vi "set_power.vi"(8 "error in (no error)":errorcluster, 10 "Power":sgl=100.0, 11 "Laser_Ethernet in":refnum<class "Laser_Ethernet.lvclass">) -> (0 "error out":errorcluster, 3 "Laser_Ethernet out":refnum<class "Laser_Ethernet.lvclass">)   [LabVIEW 2023, in "Laser_Ethernet.lvclass"]
uses:
  Laser_Ethernet.lvclass
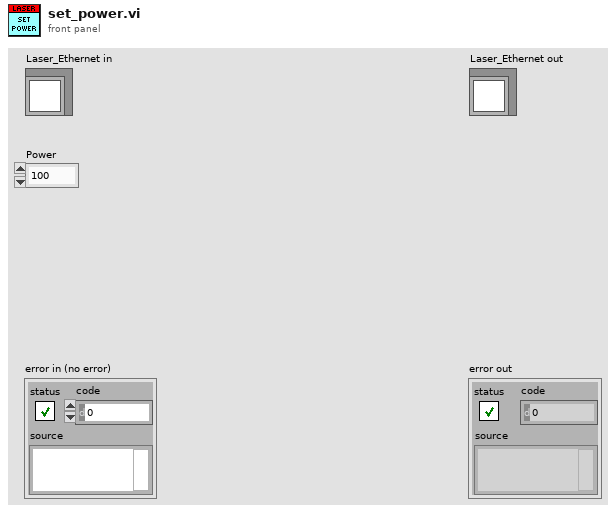
[diagram p1: front panel]
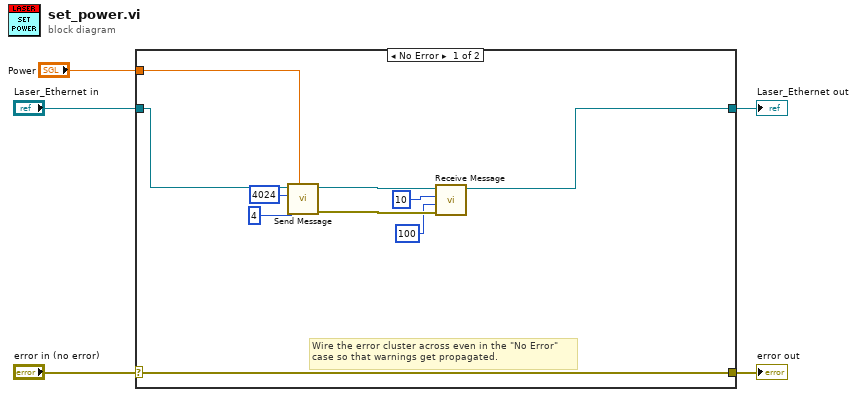
[diagram p0: block diagram]
diagram:
  n1 = case shown="No Error" "error in (no error)" {
    selector: "error in (no error)" -> [w15 w17]
    tunnel: [w15 w17] -> w4
    tunnel: [w7 w16] -> w2
    tunnel: "Laser_Ethernet in" -> [w8 w16]
    tunnel: "Power" -> [w6 _]
    frame No Error {
      # "Wire the error cluster across even in the \"No Error\"\ncase so that warnings get propagated."
      n2 = call "Send Message.vi"("Data"=w6, "Size of Data"=u32 4, "Command"=u16 4024, "object in"=w8) -> ("error out"=w11:errorcluster, "object out"=w12:refnum<class "Laser_Ethernet.lvclass">)  [unwired: 6 in]
      n3 = call "Receive Message.vi"("error in (no error)"=w11, "timeout ms (25000)"=100, "bytes to read"=10, "object in"=w12) -> ("object out"=w7:refnum<class "Laser_Ethernet.lvclass">)  [unwired: 5 in, 2 out]
    }
    frame Error {
    }
  }
  "error out" <- w4
  "Laser_Ethernet out" <- w2
